vi "tt20panel_DO_disconnect.vi"(8 "error in (no error)":errorcluster, 11 "tt20panel in":refnum<class "tt20panel.lvclass">) -> (0 "error out":errorcluster, 3 "tt20panel out":refnum<class "tt20panel.lvclass">)   [LabVIEW 2015, in "tt20panel.lvclass"]
uses:
  tt20panel.lvclass
  tt20_class/tt20.lvclass
  UI/panel_class/panel.lvclass
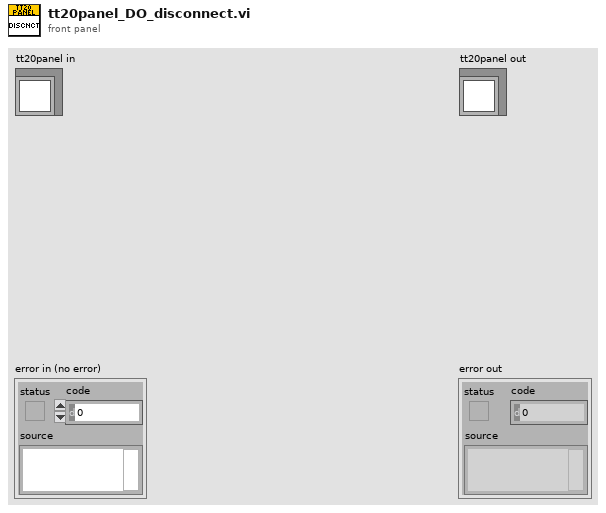
[diagram p1: front panel]
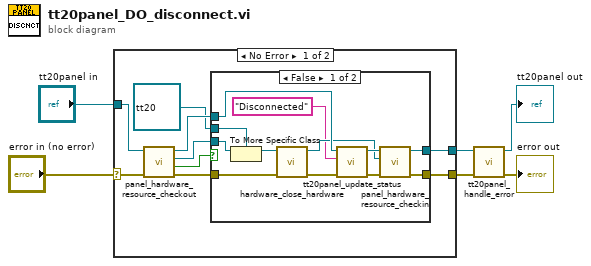
[diagram p0: block diagram]
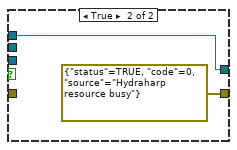
[diagram p2: hidden frame]
diagram:
  n1 = case shown="No Error" "error in (no error)" {
    selector: "error in (no error)" -> [w14 w31]
    tunnel: [w11 w31] -> w4
    tunnel: [w8 w30] -> w1
    tunnel: "tt20panel in" -> [w15 w30]
    frame No Error {
      n2 = call "panel_hardware_resource_checkout.vi"("error in (no error)"=w14, "panel in"=w15) -> ("error out"=w12:errorcluster, "timed out?"=w13:bool, "hardware.lvclass"=w9:refnum<class "hardware.lvclass">, "panel out"=w10:refnum<class "tt20panel.lvclass">)  [unwired: 6 in]
      n3 = case shown="False" w13 {
        tunnel: w12 -> [w22 _]
        tunnel: [w25 errorcluster {"status"=TRUE, "code"=0, "source"="Hydraharp resource busy"} ("error out")] -> w11
        tunnel: w10 -> [w20 w28]
        tunnel: w9 -> [w26 _]
        tunnel: refnum<class "tt20.lvclass"> refnum ("tt20.lvclass") -> [w27 _]
        tunnel: [w24 w28] -> w8
        frame False {
          n4 = To More Specific Class(target class=w27, reference=w26) -> (specific class reference=w23:refnum<class "tt20.lvclass">)  [unwired: 1 in, 1 out]
          n5 = call-dynamic "hardware_close_hardware.vi"("error in (no error)"=w22, "tt20 in"=w23) -> ("error out"=w21:errorcluster, "tt20 out"=w17:refnum<class "tt20.lvclass">)  [unwired: 8 in]
          n6 = call "tt20panel_update_status.vi"("error in (no error)"=w21, "status"="Disconnected", "tt20panel in"=w20) -> ("error out"=w18:errorcluster, "tt20panel out"=w19:refnum<class "tt20panel.lvclass">)  [unwired: 7 in]
          n7 = call "panel_hardware_resource_checkin.vi"("error in (no error)"=w18, "hardware.lvclass"=w17, "panel in"=w19) -> ("error out"=w25:errorcluster, "panel out"=w24:refnum<class "tt20panel.lvclass">)  [unwired: 7 in]
        }
        frame True {
        }
      }
    }
    frame Error {
    }
  }
  n8 = call "tt20panel_handle_error.vi"("error in (no error)"=w4, "tt20panel in"=w1) -> ("error out"=→"error out":errorcluster, "tt20panel out"=→"tt20panel out":refnum<class "tt20panel.lvclass">)  [unwired: 8 in]
